vi "Create Request Enqueuer References.vi"(8 "error in (no error)":errorcluster) -> (0 "error out":errorcluster, 1 "Launch Enqueuer":refnum<user-event>, 2 "Request-Enqueuers":T2, 3 "API-Requests":T1)   [LabVIEW 2018, in "Scripting.lvlib" / "Actor.lvlib" / "Actor.lvclass"]
uses:
  Actor.lvclass
  Request-Enqueuers.ctl
  Get State.ctl
  State.ctl
  Stop.ctl
  API-Requests.ctl
  Launch.ctl
  Interface.lvclass
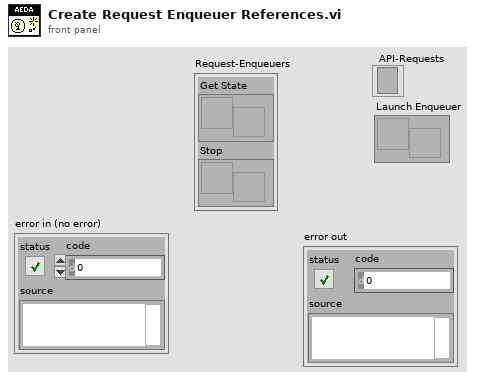
[diagram p1: front panel]
types:
  T1 = typedef "Scripting.lvlib/Actor.lvlib/Actor.lvclass/API-Requests.ctl" = refnum<event-registration>
  T2 = typedef "Scripting.lvlib/Actor.lvlib/Actor.lvclass/Request-Enqueuers.ctl" = cluster{"Get State":refnum<user-event>, "Stop":refnum<user-event>}
  T3 = typedef "Scripting.lvlib/Actor.lvlib/Actor.lvclass/Launch.ctl" = cluster{"Owner":refnum<vi>}
  T4 = typedef "Scripting.lvlib/Actor.lvlib/Interface.lvclass/Get State.ctl" = cluster{"Reply":refnum<user-event>}
  T5 = typedef "Scripting.lvlib/Actor.lvlib/Interface.lvclass/Stop.ctl" = cluster{"Type":enum16{"Normal", "Emergency"}}
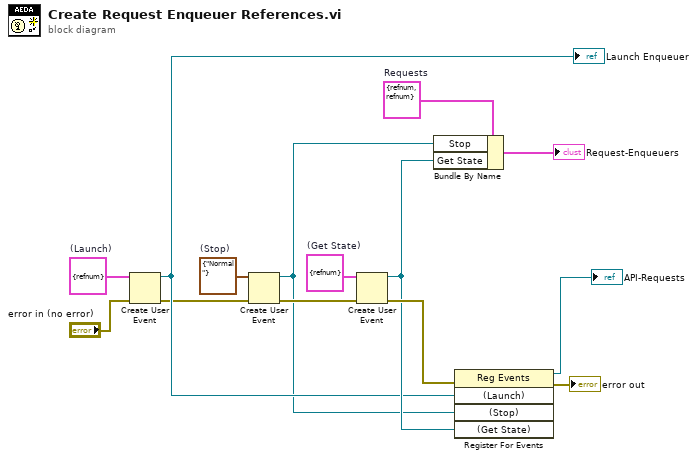
[diagram p0: block diagram]
diagram:
  w8 = T3 {"Owner"=refnum}  # (Launch)
  w10 = T4 {"Reply"=refnum}  # (Get State)
  w13 = T5 {"Type"=enum."Normal"}  # (Stop)
  w14 = T2 {"Get State"=refnum, "Stop"=refnum}  # Requests
  n1 = Create User Event(user event datatype=w8, error in="error in (no error)") -> (user event=w6:refnum<user-event>, error out=w4:errorcluster)
  "Launch Enqueuer" <- w6
  n2 = Create User Event(user event datatype=w13, error in=w4) -> (user event=w1:refnum<user-event>, error out=w3:errorcluster)
  n3 = Create User Event(user event datatype=w10, error in=w3) -> (user event=w7:refnum<user-event>, error out=w9:errorcluster)
  n4 = Bundle By Name(cluster=w14, "Stop"=w1, "Get State"=w7) -> (→"Request-Enqueuers":T2)
  n5 = register-events(error in=w9, w6, w1, w7) -> (reference out=→"API-Requests":refnum<event-registration>, error out=→"error out":errorcluster)  [unwired: 1 in]
